vi "PH_Periodic_Sequencer.PC Start.vi"(0 "i ref in":refnum<vi>, 2 "Run?":bool, 5 "error IO":errorcluster) -> (14 "i ref out":refnum<vi>, 19 "error out":errorcluster)   [LabVIEW 2014, in "PH_Periodic_Sequencer.lvlib"]
doc: "This VI sets incoming information to own attributes and GUI elements and starts or stops the procedure."
uses:
  PH_Periodic_Sequencer.lvlib
  PH_Basics/PH_Common/PH_Common.lvlib
  CS_Core/CSSystem/CSSystemLib/CSSystemLib.lvlib
  CS_Core/BaseProcess/BaseProcess.lvlib
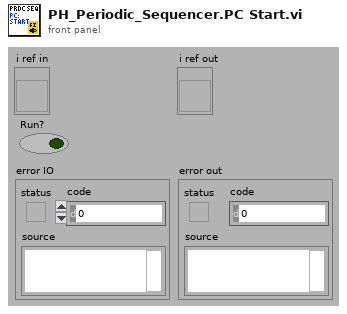
[diagram p1: front panel]
types:
  T1 = typedef "PH_Periodic_Sequencer.lvlib/PH_Periodic_Sequencer.i attribute.ctl" = cluster{"GUI Refs":cluster{"Main Off":refnum<vi>, "Start":refnum<vi>, "Ready":refnum<vi>, "Sequencer SM State":refnum<vi>, "Interval [sec]":refnum<vi>, "Wanted Shots":refnum<vi>, "Delivered Shots":refnum<vi>}, "PU Info":cluster{"Instancename":string, "State":T2, "linked":bool}[], "Sequencer":cluster{"Instancename":string, "linked?":bool, "R2S?":bool, "SM State":string}, "Run?":bool, "Interval [sec]":dbl, "PU State Refs":refnum<vi>[], "Wanted Shots":i32, "Delivered Shots":i32}
  T2 = typedef "PH_StatusHandler.lvlib/PH_StatusHandler.Status.ctl" = i16
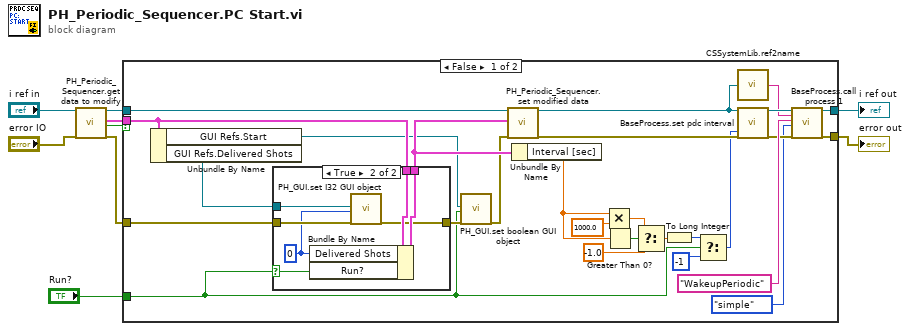
[diagram p0: block diagram]
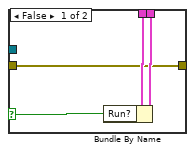
[diagram p2: hidden frame]
diagram:
  n1 = call "PH_Periodic_Sequencer.get data to modify.vi"("i ref in"="i ref in", "error in (no error)"="error IO") -> ("i ref out"=w3:refnum<vi>, "i attribute"=w8:T1, "timed out"=w7:bool, "error out"=w5:errorcluster)  [unwired: 14 in]
  n2 = case shown="False" w7 {
    tunnel: w3 -> [w36 w49]
    tunnel: [w29 w49] -> w4
    tunnel: w5 -> [w13 w48]
    tunnel: [w27 w48] -> w6
    tunnel: w8 -> [w21 _]
    tunnel: "Run?" -> [w10 _]
    frame False {
      n3 = Unbundle By Name(w21) -> ("GUI Refs.Start"=w20:refnum<vi>, "GUI Refs.Delivered Shots"=w11:refnum<vi>)
      n4 = case shown="True" w10 {
        selector: w10 -> [w40 w42]
        tunnel: [w38 w47] -> w26
        tunnel: w21 -> [w39 w46]
        tunnel: w13 -> [w37 w45]
        tunnel: [w37 w44] -> w12
        tunnel: w11 -> [_ w43]
        frame False {
          n5 = Bundle By Name(cluster=w39, "Run?"=w40) -> (w38:T1)
        }
        frame True {
          w41 = 0 ("Delivered Shots")
          n6 = Bundle By Name(cluster=w46, "Delivered Shots"=w41, "Run?"=w42) -> (w47:T1)
          n7 = call "PH_GUI.set I32 GUI object.vi"("I32 GUI Ref"=w43, "value"=w41, "error in (no error)"=w45) -> ("error out"=w44:errorcluster)  [unwired: 16 in]
        }
      }
      n8 = call "PH_GUI.set boolean GUI object.vi"("Boolean Knob GUI Ref"=w20, "Value"=w10, "error in (no error)"=w12) -> ("error out"=w19:errorcluster)  [unwired: 16 in]
      n9 = call "PH_Periodic_Sequencer.set modified data.vi"("i ref in"=w36, "i attribute"=w26, "error in (no error)"=w19) -> ("i ref out"=w30:refnum<vi>, "error out"=w28:errorcluster)  [unwired: 15 in]
      n10 = Unbundle By Name(w26) -> ("Interval [sec]"=w16:dbl)
      n11 = Multiply(x=w16, y=1000.0) -> (x*y=w15:dbl)
      n12 = Greater Than 0?(x=w16) -> (x > 0?=w18:bool)
      n13 = Select(t=w15, s=w18, f=-1.0) -> (s? t:f=w14:dbl)
      n14 = To Long Integer(number=w14) -> (32bit integer=w24:i32)
      n15 = Select(t=w24, s=w10, f=-1) -> (s? t:f=w23:i32)
      n16 = call "CSSystemLib.ref2name.vi"("obj refnum"=w30) -> ("name"=w33:string)
      n17 = call "BaseProcess.set pdc interval.vi"("i ref in"=w30, "PeriodicInterval [ms]"=w23, "error in (no error)"=w28) -> ("i ref out"=w35:refnum<vi>, "error out"=w32:errorcluster)  [unwired: 14 in, 1 out]
      n18 = call "BaseProcess.call process 1.vi"("i ref in"=w35, "Object"=w33, "Selector"="WakeupPeriodic", "CallType"=enum16{"simple", "synchronous", "asynchronous"}."simple", "error in (no error)"=w32) -> ("i ref out"=w29:refnum<vi>, "error out"=w27:errorcluster)  [unwired: 12 in, 1 out]
    }
    frame True {
    }
  }
  "error out" <- w6
  "i ref out" <- w4
